vi "AutoDrive.vi"(0 "Drive X":dbl, 5 "Drive Y":dbl, 7 "Async?":i32, 9 "Heading":dbl, 12 "X Speed":dbl, 13 "Y Speed":dbl) -> (15 "Done?":bool)   [LabVIEW 2014]
uses:
  Drivetrain Code/Drivetrain Mode.ctl
  Drivetrain Code/Drivetrain Control.ctl
  Robot Global Data.vi
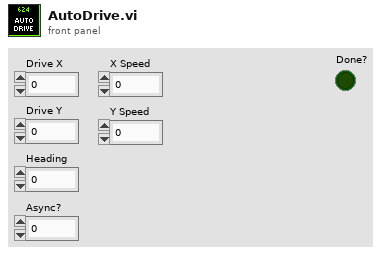
[diagram p1: front panel]
types:
  T1 = typedef "Drivetrain Control.ctl" = cluster{"Mode":T2, "Steer":dbl, "Y":dbl, "Heading Target":dbl, "Strafe X":dbl, "Y Target":dbl, "Strafe Target":dbl, "X Max Speed":dbl, "X Min Speed":dbl, "Y Max Speed":dbl, "Y Min Speed":dbl}
  T2 = typedef "Drivetrain Mode.ctl" = enum16{"Manual", "Gyro Steer", "Vision Steer", "Drive Distance"}
  T3 = typedef "Drivetrain Status.ctl" = cluster{"Y (Throttle)":sgl, "X (Steer)":sgl, "Translation X":sgl, "Center Wheel Down":bool, "Mode":T2, "Distance Drive finished?":bool, "Y Target":sgl, "X Target":sgl, "Heading Target":sgl, "Dist Drive Status":T4}
  T4 = typedef "Dist Drive Status.ctl" = cluster{"Y In Range":bool, "X In Range":bool, "Gyro In Range":bool, "Y Dist":dbl, "X Dist":dbl, "Gyro":dbl}
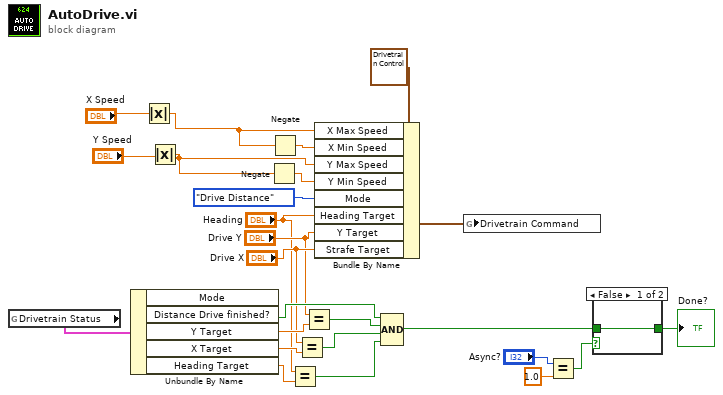
[diagram p0: block diagram]
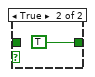
[diagram p2: hidden frame]
diagram:
  n1 = global read "Robot Global Data.vi" "Drivetrain Status"() -> (w22:T3)
  n2 = Unbundle By Name(w22) -> ("Distance Drive finished?"=w18:bool, "Y Target"=w21:sgl, "X Target"=w20:sgl, "Heading Target"=w19:sgl)  [unwired: 1 out]
  n3 = Absolute Value(x="X Speed") -> (abs(x)=w4:dbl)
  n4 = Absolute Value(x="Y Speed") -> (abs(x)=w1:dbl)
  n5 = Negate(x=w1) -> (-x=w2:dbl)
  n6 = Negate(x=w4) -> (-x=w5:dbl)
  n7 = Equal?(x="Heading", y=w19) -> (x = y?=w15:bool)
  n8 = Equal?(x="Drive X", y=w20) -> (x = y?=w16:bool)
  n9 = Equal?(x="Drive Y", y=w21) -> (x = y?=w17:bool)
  n10 = Bundle By Name(cluster=T1 {"Mode"=enum."Gyro Steer", "Steer"=0.0, "Y"=0.0, "Heading Target"=0.0, "Strafe X"=0.0, "Y Target"=0.0, "Strafe Target"=0.0, "X Max Speed"=0.0, "X Min Speed"=0.0, "Y Max Speed"=0.0, "Y Min Speed"=0.0} ("Drivetrain Command"), "X Max Speed"=w4, "X Min Speed"=w5, "Y Max Speed"=w1, "Y Min Speed"=w2, "Mode"=Drivetrain_Mode."Drive Distance", "Heading Target"="Heading", "Y Target"="Drive Y", "Strafe Target"="Drive X") -> (w25:T1)
  n11 = Compound Arithmetic op=AND(w18, w17, w16, w15) -> (w12:bool)
  n12 = global write "Robot Global Data.vi" "Drivetrain Command"(w25) -> ()
  n13 = Equal?(x="Async?", y=1.0) -> (x = y?=w10:bool)
  n14 = case shown="False" w10 {
    tunnel: w12 -> [w26 _]
    tunnel: [w26 TRUE] -> w11
    frame False {
    }
    frame True {
    }
  }
  "Done?" <- w11
